vi "Read RS232.vi"() -> ()   [LabVIEW 2014]
uses:
  <vilib>/Instr/_visa.llb/Select Event Type.ctl
  <vilib>/Instr/_visa.llb/VISA Configure Serial Port (Instr).vi
  Global Data.vi
panel:
  out "error out":errorcluster
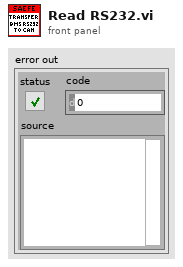
[diagram p1: front panel]
types:
  T1 = cluster{"read mode":enum16{"polling", "blocking"}, "write mode":enum16{"polling", "blocking"}}
  T2 = typedef "Select Event Type.ctl" = u32
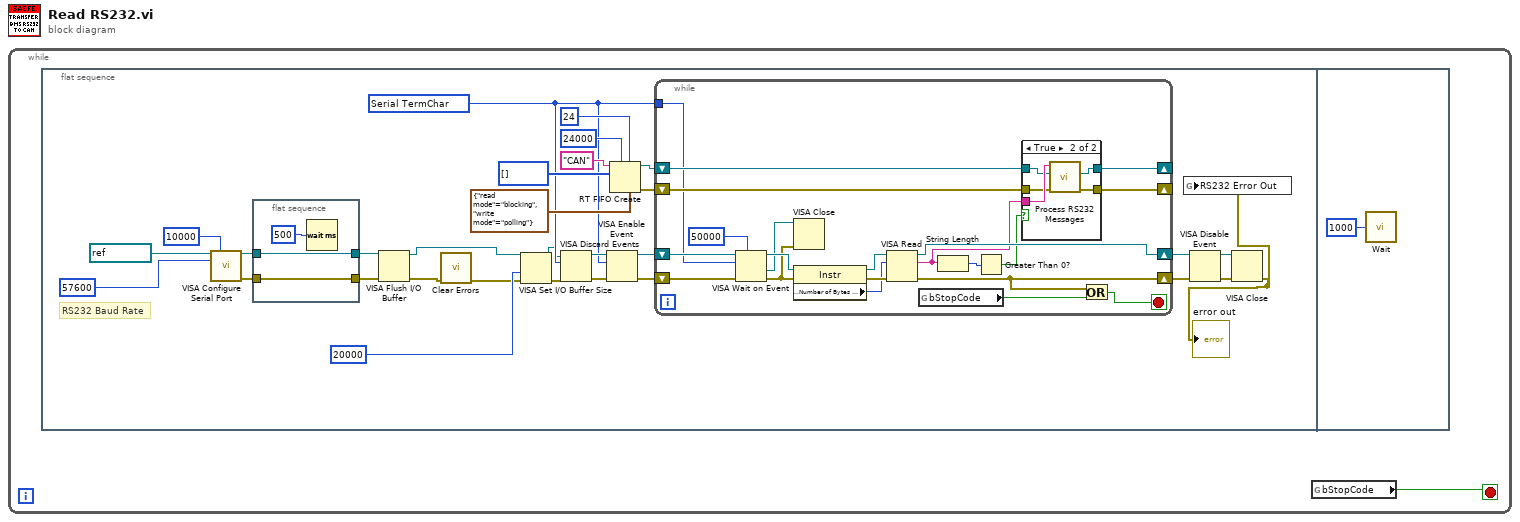
[diagram p0: block diagram]
diagram:
  n1 = while {
    stop <- w1 stop-if-true
    n2 = flat-sequence {
      frame #0 {
        w11 = T2 1073684516 items=["Service Request"=1073684491, "Trigger"=3221168138, "Clear"=1073684493, "VXI Signal"=1073684512, "VXI/VME Interrupt"=3221168161, "VXI/VME Sysfail"=1073684509, "VXI/VME Sysreset"=1073684510, "GPIB CIC"=1073684498, "GPIB Talk"=1073684499, "GPIB Listen"=1073684500, "PXI Interrupt"=1073684514, "Serial Break"=1073684515, "Serial TermChar"=1073684516, "Serial CTS"=1073684521, "Serial DSR"=1073684522, "Serial DCD"=1073684524, "Serial RI"=1073684526, "Serial Character"=1073684533, "USB Interrupt"=1073684535, "All Enabled"=1073709055] ("Event Type")
        # "RS232 Baud Rate"
        n3 = call-poly "VISA Configure Serial Port"("VISA resource name"=refnum<visa-resource-name> "COM2", "timeout (10sec)"=u32 10000, "baud rate (9600)"=u32 57600 ("Baud Rate")) -> ("VISA resource name out"=w15:refnum<visa-resource-name>, "error out"=w14:errorcluster)  [unwired: 11 in]
        n4 = flat-sequence {
          tunnel: w15 -> [w34]
          tunnel: [w34] -> w9
          tunnel: w14 -> [w33]
          tunnel: [w33] -> w8
          frame #0 {
            n5 = Wait (ms)(milliseconds to wait=u32 500) -> ()  [unwired: 1 out]
          }
        }
        n6 = VISA Flush I/O Buffer(VISA resource name=w9, error in (no error)=w8) -> (VISA resource name out=w7:refnum<visa-resource-name>, error out=w6:errorcluster)  [unwired: 1 in]
        n7 = call <vilib>:"Clear Errors.vi"("error in (no error)"=w6) -> ("error out"=w5:errorcluster)  [unwired: 5 in, 1 out]
        n8 = VISA Set I/O Buffer Size(VISA resource name=w7, size (4096)=u32 20000, error in (no error)=w5) -> (VISA resource name out=w4:refnum<visa-resource-name>, error out=w3:errorcluster)  [unwired: 1 in]
        n9 = VISA Discard Events(8:w3, 10:w11, 11:w4) -> (0:w12:errorcluster, 3:w13:refnum<visa-resource-name>)  [unwired: 1 in]
        n10 = VISA Enable Event(8:w12, 10:w11, 11:w13) -> (0:w23:errorcluster, 3:w24:refnum<visa-resource-name>)  [unwired: 1 in]
        n11 = RT FIFO Create(0:"CAN" ("name (unnamed)"), 1:u8[] [], 4:u32 24000 ("size (10)"), 6:u32 24 ("elements in array (1)"), 7:T1 {"read mode"=enum."blocking", "write mode"=enum."polling"} ("r/w modes (polling,polling)")) -> (8:w26:refnum<k33>, 11:w25:errorcluster)  [unwired: 3 in, 1 out]
        n12 = while {
          shift-right: [w49] -> _
          shift-left: w26 -> [w51]
          shift-right: [w48] -> _
          shift-left: w25 -> [w50]
          shift-right: [w37] -> w18
          shift-left: w23 -> [w46]
          shift-right: [w55] -> w22
          shift-left: w24 -> [w47]
          tunnel: w11 -> [w44]
          stop <- w35 stop-if-true
          n13 = VISA Wait on Event(7:u32 50000 ("timeout (0)"), 8:w46, 10:w44, 11:w47) -> (0:w39:errorcluster, 1:w38:refnum<visa-resource-name>, 3:w40:refnum<visa-resource-name>)  [unwired: 1 in, 1 out]
          n14 = VISA Close(VISA resource name=w38, error in (no error)=w39) -> ()  [unwired: 1 out]
          n15 = property class="Instr"(reference=w40, error in=w39) -> (reference out=w43:refnum<visa-resource-name>, error out=w42:errorcluster, "Serial Settings:Number of Bytes at Serial Port"=w41:u32)
          n16 = VISA Read(VISA resource name=w43, byte count=w41, error in (no error)=w42) -> (VISA resource name out=w55:refnum<visa-resource-name>, read buffer=w52:string, error out=w37:errorcluster)  [unwired: 1 out]
          n17 = global read "Global Data.vi" "bStopCode"() -> (w36:bool)
          n18 = String Length(string=w52) -> (length=w54:i32)
          n19 = Greater Than 0?(x=w54) -> (x > 0?=w53:bool)
          n20 = case shown="True" w53 {
            tunnel: w52 -> [_ w62]
            tunnel: w51 -> [w57 w61]
            tunnel: w50 -> [w56 w60]
            tunnel: [w57 w59] -> w49
            tunnel: [w56 w58] -> w48
            frame False {
            }
            frame True {
              n21 = call "Process RS232 Messages.vi"("error in (no error)"=w60, "rt fifo"=w61, "BMS RS232 STRING"=w62) -> ("error out"=w58:errorcluster, "rt fifo out"=w59:refnum<k33>)  [unwired: 7 in]
            }
          }
          n22 = Or(x=w37, y=w36) -> (x .or. y?=w35:bool)
        }
        n23 = VISA Disable Event(8:w18, 11:w22) -> (0:w20:errorcluster, 3:w21:refnum<visa-resource-name>)  [unwired: 2 in]
        n24 = VISA Close(VISA resource name=w21, error in (no error)=w20) -> (error out=w2:errorcluster)
        "error out" <- w2
        n25 = global write "Global Data.vi" "RS232 Error Out"(w2) -> ()
      }
      frame #1 {
        n26 = call "Wait"("Count(mSec)"=u32 1000) -> ()  [unwired: 1 out]
      }
    }
    n27 = global read "Global Data.vi" "bStopCode"() -> (w1:bool)
  }
